vi "Write Speaker Timing.vi"(8 "error in":errorcluster, 10 "spk dc":T1, 11 "PAS in":refnum<class "PAS.lvclass">=refnum) -> (0 "error out":errorcluster, 3 "PAS out":refnum<class "PAS.lvclass">)   [LabVIEW 2014]
uses:
  Switch/Switch.lvclass
  PAS.lvclass
  Controls/period_length.ctl
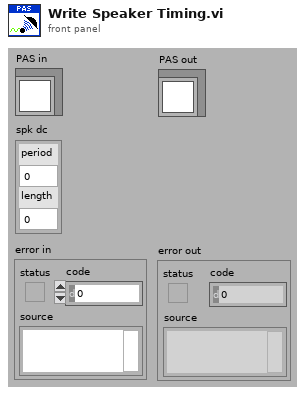
[diagram p1: front panel]
types:
  T1 = typedef "period_length.ctl" = cluster{"period":sgl, "length":sgl}
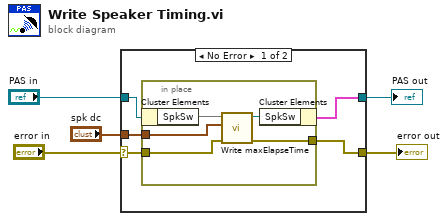
[diagram p0: block diagram]
diagram:
  n1 = case shown="No Error" "error in" {
    selector: "error in" -> [w8 w17]
    tunnel: [w7 w17] -> w4
    tunnel: [w6 w16] -> w2
    tunnel: "PAS in" -> [w10 w16]
    tunnel: "spk dc" -> [w9 _]
    frame No Error {
      n2 = in-place {
        in-place-border: w9 -> [w14]
        in-place-border: w8 -> [w13]
        in-place-border: [w12] -> w7
        n3 = in-place-cluster #1(w10) -> ("SpkSw"=w15)
        n4 = call "Write maxElapseTime.vi"("error in"=w13, "maxElapsedTime"=w14, "Switch in"=w15) -> ("error out"=w12:errorcluster, "Switch out"=w11:refnum<class "Switch.lvclass">)  [unwired: 7 in]
        n5 = in-place-cluster #1("SpkSw"=w11) -> (w6:cluster{})
      }
    }
    frame Error {
    }
  }
  "error out" <- w4
  "PAS out" <- w2
